vi "USB3 Get Usb Notification.vi"(8 "error in (no error)":errorcluster, 10 "ulTimeoutInMs":u32, 11 "pPlugNotify":T1 {"ePlugInfo" items=["ePlugged", "eUnPlugged"]}) -> (0 "error out":errorcluster, 2 "function return":i32, 3 "pPlugNotify out":T1 {"ePlugInfo" items=["ePlugged", "eUnPlugged"]})   [LabVIEW 2013, in "Octoplus_LIDAR.lvlib"]
doc: "CAMCMOSOCTUSB3_API int __cdecl USB3_GetUsbNotification(tPlugNotify * pPlugNotify, unsigned long ulTimeoutInMs);"
uses:
  <userlib>/Octoplus_LIDAR/Octoplus_LIDAR.lvlib
  <userlib>/Octoplus_LIDAR/CamCmosOctUsb3.dll
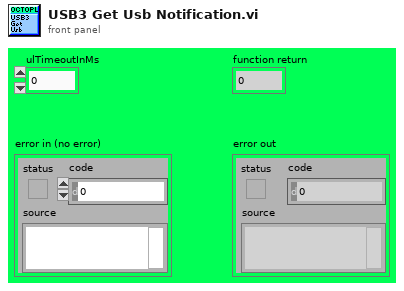
[diagram p1: front panel]
types:
  T1 = cluster{"ePlugInfo":u32, "pcCameraId[0]":i8, "pcCameraId[1]":i8, "pcCameraId[2]":i8, "pcCameraId[3]":i8, "pcCameraId[4]":i8, "pcCameraId[5]":i8, "pcCameraId[6]":i8, "pcCameraId[7]":i8, "pcCameraId[8]":i8, "pcCameraId[9]":i8, "pcCameraId[10]":i8, "pcCameraId[11]":i8, "pcCameraId[12]":i8, "pcCameraId[13]":i8, "pcCameraId[14]":i8, "pcCameraId[15]":i8, "pcCameraId[16]":i8, "pcCameraId[17]":i8, "pcCameraId[18]":i8, "pcCameraId[19]":i8, "pcCameraId[20]":i8, "pcCameraId[21]":i8, "pcCameraId[22]":i8, "pcCameraId[23]":i8, "pcCameraId[24]":i8, "pcCameraId[25]":i8, "pcCameraId[26]":i8, "pcCameraId[27]":i8, "pcCameraId[28]":i8, "pcCameraId[29]":i8, "pcCameraId[30]":i8, "pcCameraId[31]":i8, "pcCameraId[32]":i8, "pcCameraId[33]":i8, "pcCameraId[34]":i8, "pcCameraId[35]":i8, "pcCameraId[36]":i8, "pcCameraId[37]":i8, "pcCameraId[38]":i8, "pcCameraId[39]":i8, "pcCameraId[40]":i8, "pcCameraId[41]":i8, "pcCameraId[42]":i8, "pcCameraId[43]":i8, "pcCameraId[44]":i8, "pcCameraId[45]":i8, "pcCameraId[46]":i8, "pcCameraId[47]":i8, "pcCameraId[48]":i8, "pcCameraId[49]":i8, "pcCameraId[50]":i8, "pcCameraId[51]":i8, "pcCameraId[52]":i8, "pcCameraId[53]":i8, "pcCameraId[54]":i8, "pcCameraId[55]":i8, "pcCameraId[56]":i8, "pcCameraId[57]":i8, "pcCameraId[58]":i8, "pcCameraId[59]":i8, "pcCameraId[60]":i8, "pcCameraId[61]":i8, "pcCameraId[62]":i8, "pcCameraId[63]":i8, "pcCameraId[64]":i8, "pcCameraId[65]":i8, "pcCameraId[66]":i8, "pcCameraId[67]":i8, "pcCameraId[68]":i8, "pcCameraId[69]":i8, "pcCameraId[70]":i8, "pcCameraId[71]":i8, "pcCameraId[72]":i8, "pcCameraId[73]":i8, "pcCameraId[74]":i8, "pcCameraId[75]":i8, "pcCameraId[76]":i8, "pcCameraId[77]":i8, "pcCameraId[78]":i8, "pcCameraId[79]":i8, "pcCameraId[80]":i8, "pcCameraId[81]":i8, "pcCameraId[82]":i8, "pcCameraId[83]":i8, "pcCameraId[84]":i8, "pcCameraId[85]":i8, "pcCameraId[86]":i8, "pcCameraId[87]":i8, "pcCameraId[88]":i8, "pcCameraId[89]":i8, "pcCameraId[90]":i8, "pcCameraId[91]":i8, "pcCameraId[92]":i8, "pcCameraId[93]":i8, "pcCameraId[94]":i8, "pcCameraId[95]":i8, "pcCameraId[96]":i8, "pcCameraId[97]":i8, "pcCameraId[98]":i8, "pcCameraId[99]":i8, "pcCameraId[100]":i8, "pcCameraId[101]":i8, "pcCameraId[102]":i8, "pcCameraId[103]":i8, "pcCameraId[104]":i8, "pcCameraId[105]":i8, "pcCameraId[106]":i8, "pcCameraId[107]":i8, "pcCameraId[108]":i8, "pcCameraId[109]":i8, "pcCameraId[110]":i8, "pcCameraId[111]":i8, "pcCameraId[112]":i8, "pcCameraId[113]":i8, "pcCameraId[114]":i8, "pcCameraId[115]":i8, "pcCameraId[116]":i8, "pcCameraId[117]":i8, "pcCameraId[118]":i8, "pcCameraId[119]":i8, "pcCameraId[120]":i8, "pcCameraId[121]":i8, "pcCameraId[122]":i8, "pcCameraId[123]":i8, "pcCameraId[124]":i8, "pcCameraId[125]":i8, "pcCameraId[126]":i8, "pcCameraId[127]":i8, "pcCameraId[128]":i8, "pcCameraId[129]":i8, "pcCameraId[130]":i8, "pcCameraId[131]":i8, "pcCameraId[132]":i8, "pcCameraId[133]":i8, "pcCameraId[134]":i8, "pcCameraId[135]":i8, "pcCameraId[136]":i8, "pcCameraId[137]":i8, "pcCameraId[138]":i8, "pcCameraId[139]":i8, "pcCameraId[140]":i8, "pcCameraId[141]":i8, "pcCameraId[142]":i8, "pcCameraId[143]":i8, "pcCameraId[144]":i8, "pcCameraId[145]":i8, "pcCameraId[146]":i8, "pcCameraId[147]":i8, "pcCameraId[148]":i8, "pcCameraId[149]":i8, "pcCameraId[150]":i8, "pcCameraId[151]":i8, "pcCameraId[152]":i8, "pcCameraId[153]":i8, "pcCameraId[154]":i8, "pcCameraId[155]":i8, "pcCameraId[156]":i8, "pcCameraId[157]":i8, "pcCameraId[158]":i8, "pcCameraId[159]":i8, "pcCameraId[160]":i8, "pcCameraId[161]":i8, "pcCameraId[162]":i8, "pcCameraId[163]":i8, "pcCameraId[164]":i8, "pcCameraId[165]":i8, "pcCameraId[166]":i8, "pcCameraId[167]":i8, "pcCameraId[168]":i8, "pcCameraId[169]":i8, "pcCameraId[170]":i8, "pcCameraId[171]":i8, "pcCameraId[172]":i8, "pcCameraId[173]":i8, "pcCameraId[174]":i8, "pcCameraId[175]":i8, "pcCameraId[176]":i8, "pcCameraId[177]":i8, "pcCameraId[178]":i8, "pcCameraId[179]":i8, "pcCameraId[180]":i8, "pcCameraId[181]":i8, "pcCameraId[182]":i8, "pcCameraId[183]":i8, "pcCameraId[184]":i8, "pcCameraId[185]":i8, "pcCameraId[186]":i8, "pcCameraId[187]":i8, "pcCameraId[188]":i8, "pcCameraId[189]":i8, "pcCameraId[190]":i8, "pcCameraId[191]":i8, "pcCameraId[192]":i8, "pcCameraId[193]":i8, "pcCameraId[194]":i8, "pcCameraId[195]":i8, "pcCameraId[196]":i8, "pcCameraId[197]":i8, "pcCameraId[198]":i8, "pcCameraId[199]":i8, "pcCameraId[200]":i8, "pcCameraId[201]":i8, "pcCameraId[202]":i8, "pcCameraId[203]":i8, "pcCameraId[204]":i8, "pcCameraId[205]":i8, "pcCameraId[206]":i8, "pcCameraId[207]":i8, "pcCameraId[208]":i8, "pcCameraId[209]":i8, "pcCameraId[210]":i8, "pcCameraId[211]":i8, "pcCameraId[212]":i8, "pcCameraId[213]":i8, "pcCameraId[214]":i8, "pcCameraId[215]":i8, "pcCameraId[216]":i8, "pcCameraId[217]":i8, "pcCameraId[218]":i8, "pcCameraId[219]":i8, "pcCameraId[220]":i8, "pcCameraId[221]":i8, "pcCameraId[222]":i8, "pcCameraId[223]":i8, "pcCameraId[224]":i8, "pcCameraId[225]":i8, "pcCameraId[226]":i8, "pcCameraId[227]":i8, "pcCameraId[228]":i8, "pcCameraId[229]":i8, "pcCameraId[230]":i8, "pcCameraId[231]":i8, "pcCameraId[232]":i8, "pcCameraId[233]":i8, "pcCameraId[234]":i8, "pcCameraId[235]":i8, "pcCameraId[236]":i8, "pcCameraId[237]":i8, "pcCameraId[238]":i8, "pcCameraId[239]":i8, "pcCameraId[240]":i8, "pcCameraId[241]":i8, "pcCameraId[242]":i8, "pcCameraId[243]":i8, "pcCameraId[244]":i8, "pcCameraId[245]":i8, "pcCameraId[246]":i8, "pcCameraId[247]":i8, "pcCameraId[248]":i8, "pcCameraId[249]":i8, "pcCameraId[250]":i8, "pcCameraId[251]":i8, "pcCameraId[252]":i8, "pcCameraId[253]":i8, "pcCameraId[254]":i8, "pcCameraId[255]":i8, "pcCameraId[256]":i8, "pcCameraId[257]":i8, "pcCameraId[258]":i8, "pcCameraId[259]":i8}
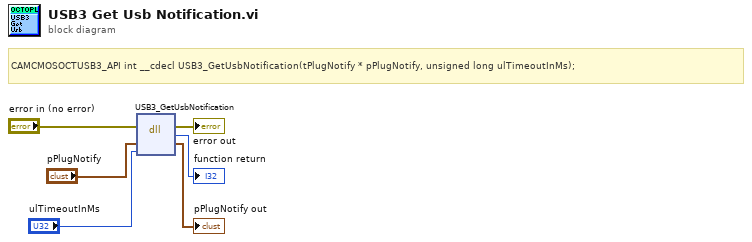
[diagram p0: block diagram]
diagram:
  # "CAMCMOSOCTUSB3_API int __cdecl USB3_GetUsbNotification(tPlugNotify * pPlugNotify, unsigned long ulTimeoutInMs);"
  n1 = dll-call lib="C:/Program Files/National Instruments/LabVIEW 2013/user.lib/Octoplus_LIDAR/CamCmosOctUsb3.*" fn="USB3_GetUsbNotification"(error in="error in (no error)", "pPlugNotify"="pPlugNotify", "ulTimeoutInMs"="ulTimeoutInMs") -> (error out=→"error out":errorcluster, →"function return":i32, "pPlugNotify"=→"pPlugNotify out":T1)  [unwired: 3 in, 1 out]
